vi "DEAD_BAND.vi"(10 "axis input":dbl, 11 "deadband input":dbl) -> (3 "axis output":dbl)   [LabVIEW 2014]
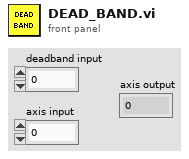
[diagram p1: front panel]
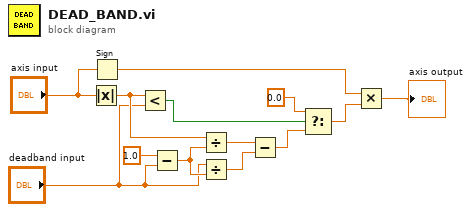
[diagram p0: block diagram]
diagram:
  n1 = Absolute Value(x="axis input") -> (abs(x)=w4:dbl)
  n2 = Sign(1:"axis input") -> (0:w10:dbl)
  n3 = Less?(x=w4, y="deadband input") -> (x < y?=w8:bool)
  n4 = Subtract(x=1.0, y="deadband input") -> (x-y=w3:dbl)
  n5 = Divide(x=w4, y=w3) -> (x/y=w6:dbl)
  n6 = Divide(x="deadband input", y=w3) -> (x/y=w5:dbl)
  n7 = Subtract(x=w6, y=w5) -> (x-y=w7:dbl)
  n8 = Select(t=0.0, s=w8, f=w7) -> (s? t:f=w12:dbl)
  n9 = Multiply(x=w10, y=w12) -> (x*y=→"axis output":dbl)
